vi "display queue contents.vi"(8 "show queue contents":bool=TRUE, 9 "Queue":enum16{"Message", "Comms", "Data"}(ring), 10 "Queues":T1) -> (2 "Array 2":string[](array[string]), 3 "Queue lengths":i32[](array[numeric]))   [LabVIEW 2018]
uses:
  Type Defs/Queues cluster.ctl
  ICL-LabVIEW_General/Message Scheduler/message scheduler.lvclass
  <vilib>/ErrorRing/Error Ring.xnode
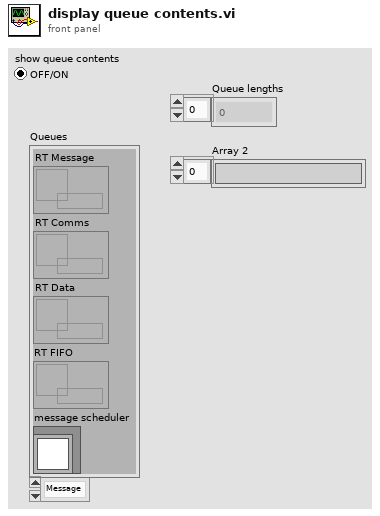
[diagram p1: front panel]
types:
  T1 = typedef "Queues cluster.ctl" = cluster{"RT Message":refnum<queue>, "RT Comms":refnum<queue>, "RT Data":refnum<queue>, "RT FIFO":refnum<queue>, "message scheduler":refnum<class "message scheduler.lvclass">}
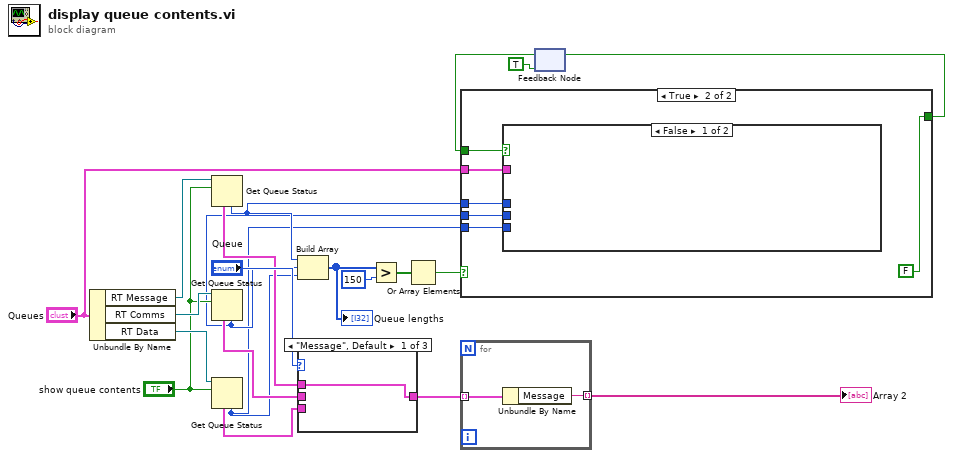
[diagram p0: block diagram]
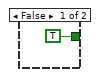
[diagram p2: hidden frame]
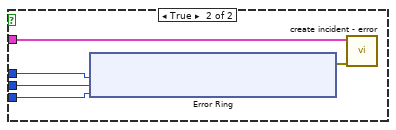
[diagram p3: hidden frame]
diagram:
  n1 = Unbundle By Name("Queues") -> ("RT Message"=w19:refnum<queue>, "RT Comms"=w17:refnum<queue>, "RT Data"=w18:refnum<queue>)
  n2 = Get Queue Status(queue=w19, return elements? (F)="show queue contents") -> (# elements in queue=w8:i32, elements=w13:cluster{"Message":string, "Data":variant}[])  [unwired: 1 in, 6 out]
  n3 = Get Queue Status(queue=w17, return elements? (F)="show queue contents") -> (# elements in queue=w7:i32, elements=w14:cluster{"Message":string, "Data":variant}[])  [unwired: 1 in, 6 out]
  n4 = Get Queue Status(queue=w18, return elements? (F)="show queue contents") -> (# elements in queue=w6:i32, elements=w16:cluster{"Message":string, "Data":variant}[])  [unwired: 1 in, 6 out]
  n5 = Build Array(w8, w7, w6) -> (w11:i32[])
  "Queue lengths" <- w11
  n6 = case shown="\"Message\", Default" "Queue" {
    tunnel: w16 -> [_ _ w24]
    tunnel: w14 -> [_ w23 _]
    tunnel: w13 -> [w22 _ _]
    tunnel: [w22 w23 w24] -> w12
    frame "Message", Default {
    }
    frame "Comms" {
    }
    frame "Data" {
    }
  }
  n7 = Greater?(x=w11, y=150) -> (0:w9:bool[])
  n8 = Or Array Elements(Boolean array=w9) -> (logical OR=w2:bool)
  n9 = for {
    tunnel: w12 -> [w26] mode=indexing
    tunnel: [w25] -> w20 mode=indexing
    n10 = Unbundle By Name(w26) -> ("Message"=w25:string)
  }
  "Array 2" <- w20
  n11 = feedback #1(TRUE) -> (w1:bool)
  n12 = case shown="True" w2 {
    tunnel: w8 -> [_ w33]
    tunnel: w7 -> [_ w32]
    tunnel: w6 -> [_ w31]
    tunnel: "Queues" -> [_ w30]
    tunnel: [TRUE FALSE] -> w4
    tunnel: w1 -> [_ w29]
    frame False {
    }
    frame True {
      n13 = case shown="False" w29 {
        tunnel: w33 -> [_ w37]
        tunnel: w32 -> [_ w36]
        tunnel: w31 -> [_ w35]
        tunnel: w30 -> [_ w34]
        frame False {
        }
        frame True {
          n14 = xnode "Error Ring"("parameter 0"=w37, "parameter 1"=w36, "parameter 2"=w35) -> ("error out"=w38:errorcluster)
          n15 = call "create incident - error.vi"("error"=w38, "RT Queues"=w34) -> ()  [unwired: 9 in, 1 out]
        }
      }
    }
  }
  n16 = feedback-in #1(w4) -> ()
